vi "zmq_recv_event.vi"(4 "error in":errorcluster, 5 "timeout (none)":i32=-1, 6 "sockets":refnum<class "Socket.lvclass">[](array[class]), 7 "poll event":refnum<user-event>) -> (0 "error out":errorcluster, 3 "poll event out":refnum<user-event>)   [LabVIEW 2025, in "ZeroMQ.lvlib" / "Socket.lvclass"]
doc: "Poll several sockets for input, and generate events when they receive data. This data can then be retrieved through an Event Structure.\n\nChecks whether each socket in <b>sockets</b> has data ready to receive, receives the data and raises an event. If no events happen within <b>timeout</b>, returns.\n\nIt is probably unsafe to use a <b>timeout</b> of 0, as if no data is received on any of the sockets, the LabVIEW process will hang indefinitely.\n\nMore details: http://sourceforge.net/p/labview-zmq/wiki/PollingAndEvents/"
uses:
  Socket.lvclass
  poll_event_data.ctl
  socket_options.ctl
  poll_type.ctl
  zmq_poll_scalar.vi
  ZeroMQ.lvlib
panel:
  # "ØMQ"
  # "labview"
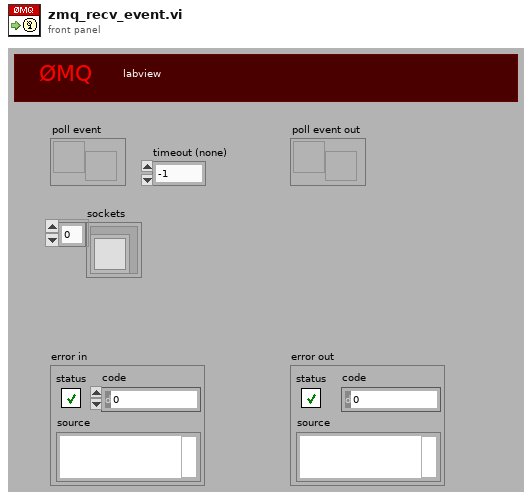
[diagram p1: front panel]
types:
  T1 = typedef "ZeroMQ.lvlib/socket_options.ctl" = enum8{"NONE", "ZMQ_HWM", "<2>", "ZMQ_SWAP", "ZMQ_AFFINITY", "ZMQ_ROUTING_ID", "ZMQ_SUBSCRIBE", "ZMQ_UNSUBSCRIBE", "ZMQ_RATE", "ZMQ_RECOVERY_IVL", "ZMQ_MCAST_LOOP", "ZMQ_SNDBUF", "ZMQ_RCVBUF", "ZMQ_RCVMORE", "ZMQ_FD", "ZMQ_EVENTS", "ZMQ_TYPE", "ZMQ_LINGER", "ZMQ_RECONNECT_IVL", "ZMQ_BACKLOG", "ZMQ_RECOVERY_IVL_MSEC", "ZMQ_RECONNECT_IVL_MAX", "ZMQ_MAXMSGSIZE", "ZMQ_SNDHWM", "ZMQ_RCVHWM", "ZMQ_MULTICAST_HOPS", "<26>", "ZMQ_RCVTIMEO", "ZMQ_SNDTIMEO", "<29>", "<30>", "ZMQ_IPV4ONLY", "ZMQ_LAST_ENDPOINT", "ZMQ_ROUTER_MANDATORY", "ZMQ_TCP_KEEPALIVE", "ZMQ_TCP_KEEPALIVE_CNT", "ZMQ_TCP_KEEPALIVE_IDLE", "ZMQ_TCP_KEEPALIVE_INTVL", "ZMQ_TCP_ACCEPT_FILTER", "ZMQ_IMMEDIATE", "ZMQ_XPUB_VERBOSE", "ZMQ_ROUTER_RAW", "ZMQ_IPV6", "ZMQ_MECHANISM", "ZMQ_PLAIN_SERVER", "ZMQ_PLAIN_USERNAME", "ZMQ_PLAIN_PASSWORD", "ZMQ_CURVE_SERVER", "ZMQ_CURVE_PUBLICKEY", "ZMQ_CURVE_SECRETKEY", "ZMQ_CURVE_SERVERKEY", "ZMQ_PROBE_ROUTER", "ZMQ_REQ_CORRELATE", "ZMQ_REQ_RELAXED", "ZMQ_CONFLATE", "ZMQ_ZAP_DOMAIN", "ZMQ_ROUTER_HANDOVER", "ZMQ_TOS", "ZMQ_IPC_FILTER_PID", "ZMQ_IPC_FILTER_UID", "ZMQ_IPC_FILTER_GID", "ZMQ_CONNECT_ROUTING_ID", "ZMQ_GSSAPI_SERVER", "ZMQ_GSSAPI_PRINCIPAL", "ZMQ_GSSAPI_SERVICE_PRINCIPAL", "ZMQ_GSSAPI_PLAINTEXT", "ZMQ_HANDSHAKE_IVL", "<67>", "ZMQ_SOCKS_PROXY", "ZMQ_XPUB_NODROP", "ZMQ_BLOCKY", "ZMQ_XPUB_MANUAL", "ZMQ_XPUB_WELCOME_MSG", "ZMQ_STREAM_NOTIFY", "ZMQ_INVERT_MATCHING", "ZMQ_HEARTBEAT_IVL", "ZMQ_HEARTBEAT_TTL", "ZMQ_HEARTBEAT_TIMEOUT", "ZMQ_XPUB_VERBOSER", "ZMQ_CONNECT_TIMEOUT", "ZMQ_TCP_MAXRT", "ZMQ_THREAD_SAFE", "<82>", "<83>", "ZMQ_MULTICAST_MAXTPDU", "ZMQ_VMCI_BUFFER_SIZE", "ZMQ_VMCI_BUFFER_MIN_SIZE", "ZMQ_VMCI_BUFFER_MAX_SIZE", "ZMQ_VMCI_CONNECT_TIMEOUT", "ZMQ_USE_FD", "ZMQ_GSSAPI_PRINCIPAL_NAMETYPE", "ZMQ_GSSAPI_SERVICE_PRINCIPAL_NAMETYPE", "ZMQ_BINDTODEVICE", "ZMQ_ZAP_ENFORCE_DOMAIN", "ZMQ_LOOPBACK_FASTPATH", "ZMQ_METADATA", "ZMQ_MULTICAST_LOOP", "ZMQ_ROUTER_NOTIFY"}
  T2 = typedef "ZeroMQ.lvlib/poll_type.ctl" = enum16{"None", "In", "Out", "In/Out"}
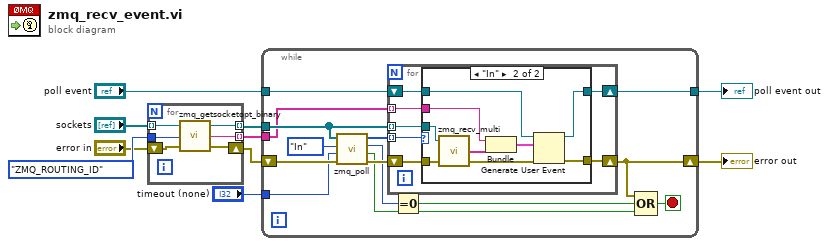
[diagram p0: block diagram]
diagram:
  n1 = for {
    tunnel: "sockets" -> [w16] mode=indexing
    tunnel: socket_options."ZMQ_ROUTING_ID" ("option") -> [w15]
    shift-right: [w13] -> w3
    shift-left: "error in" -> [w14]
    tunnel: [w12] -> w1 mode=indexing
    tunnel: [w11] -> w4 mode=indexing
    n2 = call "zmq_getsocketopt_binary.vi"("error in"=w14, "option"=w15, "socket in"=w16) -> ("error out"=w13:errorcluster, "value"=w12:string, "socket out"=w11:refnum<class "Socket.lvclass">)
  }
  n3 = while {
    tunnel: w4 -> [w30]
    tunnel: "poll event" -> [w29]
    tunnel: [w28] -> w8
    shift-right: [w17] -> w10
    shift-left: w3 -> [w27]
    tunnel: "timeout (none)" -> [w20]
    tunnel: w1 -> [w18]
    stop <- w24 stop-if-true
    n4 = call-poly "zmq_poll.vi"("error in"=w27, "timeout"=w20, "poll type"=poll_type."In", "sockets"=w30) -> ("error out"=w26:errorcluster, "timed out?"=w19:bool, "nevents"=w25:i32, "polled events"=w21:T2[])
    n5 = for {
      shift-right: [w36] -> w28
      shift-left: w29 -> [w37]
      shift-right: [w34] -> w17
      shift-left: w26 -> [w35]
      tunnel: w30 -> [w33] mode=indexing
      tunnel: w21 -> [w32] mode=indexing
      tunnel: w18 -> [w31] mode=indexing
      n6 = case shown="\"In\"" w32 {
        tunnel: w37 -> [w39 w48]
        tunnel: [w39 w47] -> w36
        tunnel: w35 -> [w38 w46]
        tunnel: [w38 w45] -> w34
        tunnel: w33 -> [_ w44]
        tunnel: w31 -> [_ w40]
        frame Default {
        }
        frame "In" {
          n7 = call "zmq_recv_multi.vi"("error in"=w46, "socket in"=w44) -> ("error out"=w41:errorcluster, "parts"=w42:string[])  [unwired: 1 in, 1 out]
          n8 = Bundle("value"=w40, "parts"=w42) -> (w43:cluster{"value":string, "parts":string[]})  [unwired: 1 in]
          n9 = Generate User Event(user event=w48, event data cluster=w43, error in=w41) -> (user event out=w47:refnum<user-event>, error out=w45:errorcluster)  [unwired: 1 in]
        }
      }
    }
    n10 = Equal To 0?(x=w25) -> (x = 0?=w23:bool)
    n11 = Compound Arithmetic op=OR(w17, w23, w19) -> (w24:bool)
  }
  "error out" <- w10
  "poll event out" <- w8
